vi "Save Results To Disk.vi"(0 "Save To Path":path, 1 "Sample Name":string, 2 "User Name":string, 3 "Test Date":string, 5 "Test Settings":T2={"Current Level"=0.0, "Compliance Level"=0.0, "Soak Time"=0.0, "NPLC Voltmeter"=1.0, "Count Voltmeter"=1, "NPLC Ammeter"=1.0, "Count Ammeter"=1, "Sample Resistivity"=enum."Low", "Sample Thickness"=0.0, "Magnetic Flux"=0.0, "Units"=enum."T", "Sample Dimensions x"=0.0, "Sample Dimensions y"=0.0, "Sample Dimensions D1"=0.0, "Sample Dimensions D2"=0.0, "Sample Width Ws"=0.0, "Slot Number of 3765 Card"=1} {"Slot Number of 3765 Card" min=1 max=6 step=1; "NPLC Ammeter" min=0.01 max=10.0; "NPLC Voltmeter" min=0.01 max=10.0 format="%^#_6g"; "Count Ammeter" min=1 max=1024; "Count Voltmeter" min=1 max=1024; "Soak Time" format="%^#_6g"; "Compliance Level" format="%^#_6g"; "Current Level" format="%^#_6e"}, 7 "Van Der Pauw Measurements":T5, 9 "Van Der Pauw Resistance Results":T3, 11 "error in (no error)":errorcluster, 12 "Hall Measurements":T5, 13 "Hall Effect Results":T4) -> (15 "error out":errorcluster)   [LabVIEW 2016]
uses:
  Hall Effect Library/Public/Controls/Resisitivity.ctl
  Hall Effect Library/Hall Effect Library.lvlib
panel:
  # "NPLC"
  # "A"
  # "V"
  # "s"
  # "Measure Count"
  # "cm"
  # "cm"
  # "cm"
  # "cm"
  # "cm"
  # "cm"
  # "Geometric Factor"
  # "Resistance Ratio"
  # "Resistivity"
  # "Ohm cm"
  # "Ohm cm"
  # "Ohm cm"
  # "Hall Coefficient"
  # "cm^2/V s"
  # "Ohm cm"
  # "cm^-3"
  # "Ohm cm"
  # "Ohm cm"
  # "Current"
  # "Pos"
  # "Volts"
  # "Neg"
  # "Direction"
  # "Magnet"
  # "Pos"
  # "Volts"
  # "Neg"
  # "Polarity"
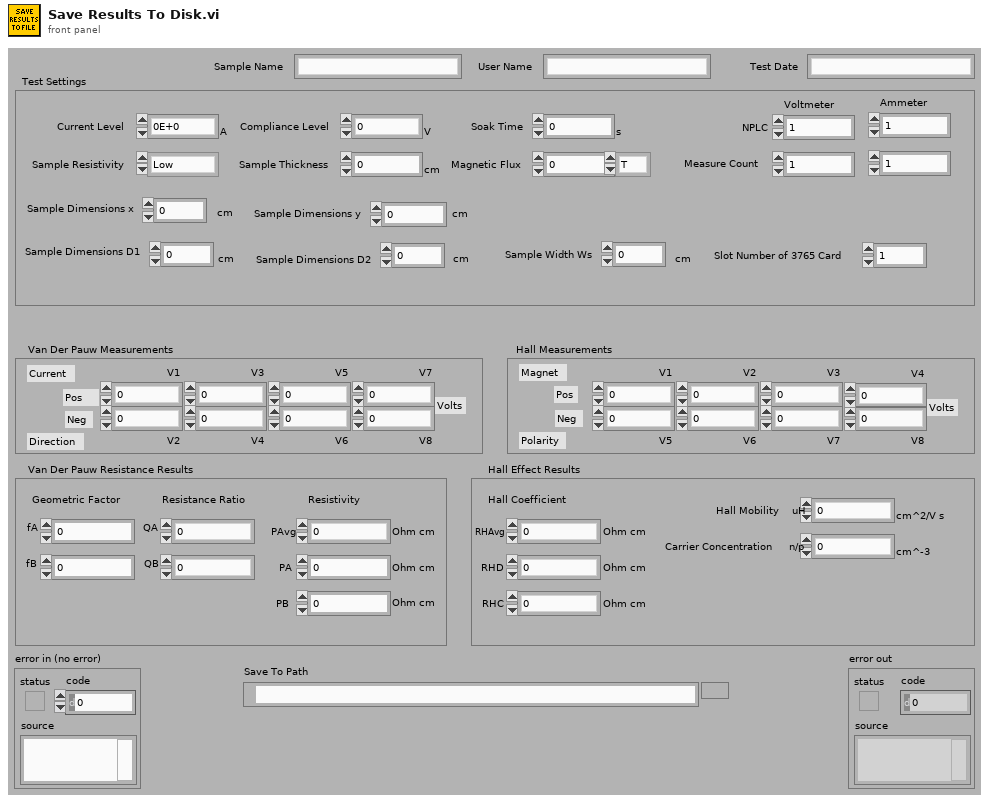
[diagram p1: front panel]
types:
  T1 = typedef "Hall Effect Library.lvlib/Resisitivity.ctl" = enum16{"Low", "High"}
  T2 = cluster{"Current Level":dbl, "Compliance Level":dbl, "Soak Time":dbl, "NPLC Voltmeter":dbl, "Count Voltmeter":i32, "NPLC Ammeter":dbl, "Count Ammeter":i32, "Sample Resistivity":T1, "Sample Thickness":dbl, "Magnetic Flux":dbl, "Units":enum16{"Gs", "T"}, "Sample Dimensions x":dbl, "Sample Dimensions y":dbl, "Sample Dimensions D1":dbl, "Sample Dimensions D2":dbl, "Sample Width Ws":dbl, "Slot Number of 3765 Card":u8}
  T3 = cluster{"fA":dbl, "fB":dbl, "QA":dbl, "QB":dbl, "PAvg":dbl, "PA":dbl, "PB":dbl}
  T4 = cluster{"RHD":dbl, "RHC":dbl, "RHAvg":dbl, "uH":dbl, "n/p":dbl}
  T5 = cluster{"V1":dbl, "V2":dbl, "V3":dbl, "V4":dbl, "V5":dbl, "V6":dbl, "V7":dbl, "V8":dbl}
  T6 = enum16{"open", "replace", "create", "open or create", "replace or create", "replace or create with confirmation"}
  T7 = cluster{"Van Der Pauw Currents[0]":dbl, "Van Der Pauw Currents[1]":dbl, "Van Der Pauw Currents[2]":dbl, "Van Der Pauw Currents[3]":dbl, "Van Der Pauw Currents[4]":dbl, "Van Der Pauw Currents[5]":dbl, "Van Der Pauw Currents[6]":dbl, "Van Der Pauw Currents[7]":dbl}
  T8 = cluster{"Hall Effect Currents[0]":dbl, "Hall Effect Currents[1]":dbl, "Hall Effect Currents[2]":dbl, "Hall Effect Currents[3]":dbl, "Hall Effect Currents[4]":dbl, "Hall Effect Currents[5]":dbl, "Hall Effect Currents[6]":dbl, "Hall Effect Currents[7]":dbl}
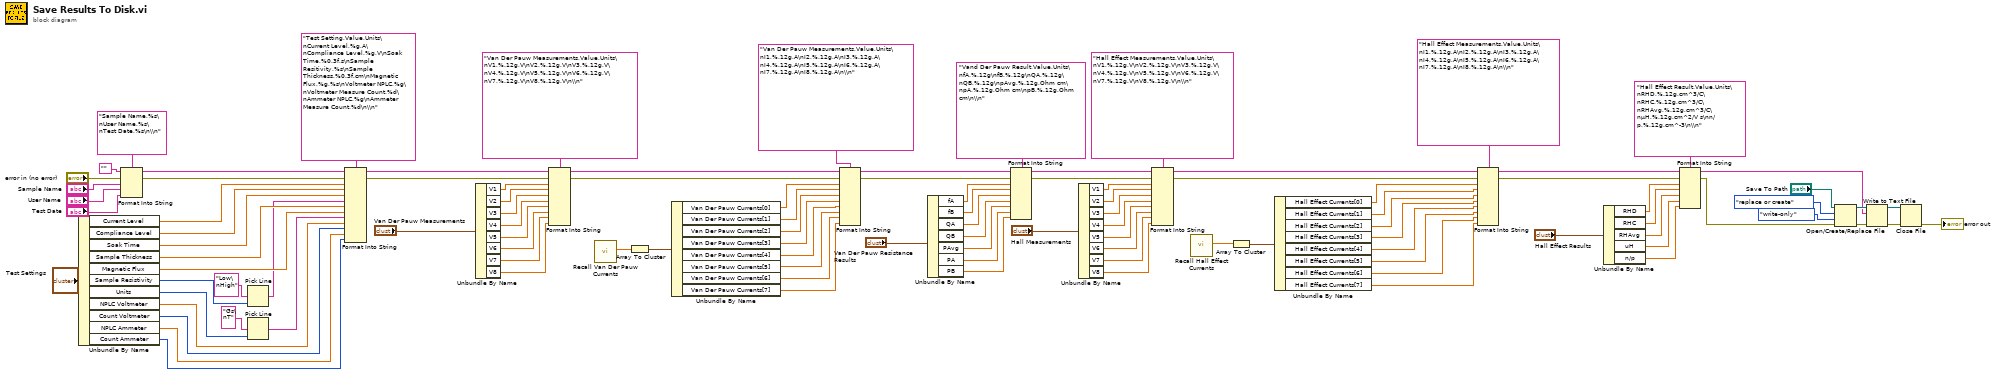
[diagram p0: block diagram]
diagram:
  n1 = Unbundle By Name("Test Settings") -> ("Current Level"=w98:dbl, "Compliance Level"=w97:dbl, "Soak Time"=w96:dbl, "Sample Thickness"=w95:dbl, "Magnetic Flux"=w94:dbl, "Sample Resistivity"=w90:T1, "Units"=w91:enum16{"Gs", "T"}, "NPLC Voltmeter"=w35:dbl, "Count Voltmeter"=w34:i32, "NPLC Ammeter"=w33:dbl, "Count Ammeter"=w32:i32)
  n2 = Format Into String(format string="Sample Name,%s\nUser Name,%s\nTest Date,%s\n\\n", initial string="", error in="error in (no error)", "Sample Name", "User Name", "Test Date") -> (resulting string=w86:string, error out=w87:errorcluster)
  n3 = Pick Line(multi-line string="Low\nHigh", line index=w90) -> (output string=w89:string)  [unwired: 1 out]
  n4 = Pick Line(multi-line string="Gs\nT", line index=w91) -> (output string=w88:string)  [unwired: 1 out]
  n5 = Format Into String(format string="Test Setting,Value,Units\nCurrent Level,%g,A\nCompliance Level,%g,V\nSoak Time,%0.3f,s\nSample Resitivity,%s\nSample Thickness,%0.3f,cm\nMagnetic Flux,%g,%s\nVoltmeter NPLC,%g\nVoltmeter Measure Count,%d\nAmmeter NPLC,%g\nAmmeter Measure Count,%d\n\\n", initial string=w86, error in=w87, w98, w97, w96, w89, w95, w94, w88, w35, w34, w33, w32) -> (resulting string=w83:string, error out=w82:errorcluster)
  n6 = Unbundle By Name("Van Der Pauw Measurements") -> ("V1"=w81:dbl, "V2"=w80:dbl, "V3"=w79:dbl, "V4"=w78:dbl, "V5"=w77:dbl, "V6"=w76:dbl, "V7"=w75:dbl, "V8"=w74:dbl)
  n7 = Format Into String(format string="Van Der Pauw Measurements,Value,Units\nV1,%.12g,V\nV2,%.12g,V\nV3,%.12g,V\nV4,%.12g,V\nV5,%.12g,V\nV6,%.12g,V\nV7,%.12g,V\nV8,%.12g,V\n\\n", initial string=w83, error in=w82, w81, w80, w79, w78, w77, w76, w75, w74) -> (resulting string=w28:string, error out=w27:errorcluster)
  n8 = call "Recall Van Der Pauw Currents.vi"() -> ("Van Der Pauw Currents"=w30:dbl[])  [unwired: 11 in]
  n9 = Array To Cluster(array=w30) -> (cluster=w29:T7)
  n10 = Unbundle By Name(w29) -> ("Van Der Pauw Currents[0]"=w26:dbl, "Van Der Pauw Currents[1]"=w25:dbl, "Van Der Pauw Currents[2]"=w24:dbl, "Van Der Pauw Currents[3]"=w23:dbl, "Van Der Pauw Currents[4]"=w22:dbl, "Van Der Pauw Currents[5]"=w21:dbl, "Van Der Pauw Currents[6]"=w20:dbl, "Van Der Pauw Currents[7]"=w19:dbl)
  n11 = Format Into String(format string="Van Der Pauw Measurements,Value,Units\nI1,%.12g,A\nI2,%.12g,A\nI3,%.12g,A\nI4,%.12g,A\nI5,%.12g,A\nI6,%.12g,A\nI7,%.12g,A\nI8,%.12g,A\n\\n", initial string=w28, error in=w27, w26, w25, w24, w23, w22, w21, w20, w19) -> (resulting string=w17:string, error out=w16:errorcluster)
  n12 = Unbundle By Name("Van Der Pauw Resistance Results") -> ("fA"=w62:dbl, "fB"=w61:dbl, "QA"=w60:dbl, "QB"=w59:dbl, "PAvg"=w58:dbl, "PA"=w57:dbl, "PB"=w56:dbl)
  n13 = Format Into String(format string="Vand Der Pauw Result,Value,Units\nfA,%.12g\nfB,%.12g\nQA,%.12g\nQB,%.12g\npAvg,%.12g,Ohm cm\npA,%.12g,Ohm cm\npB,%.12g,Ohm cm\n\\n", initial string=w17, error in=w16, w62, w61, w60, w59, w58, w57, w56) -> (resulting string=w55:string, error out=w54:errorcluster)
  n14 = Unbundle By Name("Hall Measurements") -> ("V1"=w66:dbl, "V2"=w67:dbl, "V3"=w68:dbl, "V4"=w69:dbl, "V5"=w70:dbl, "V6"=w71:dbl, "V7"=w72:dbl, "V8"=w73:dbl)
  n15 = Format Into String(format string="Hall Effect Measurements,Value,Units\nV1,%.12g,V\nV2,%.12g,V\nV3,%.12g,V\nV4,%.12g,V\nV5,%.12g,V\nV6,%.12g,V\nV7,%.12g,V\nV8,%.12g,V\n\\n", initial string=w55, error in=w54, w66, w67, w68, w69, w70, w71, w72, w73) -> (resulting string=w13:string, error out=w12:errorcluster)
  n16 = call "Recall Hall Effect Currents.vi"() -> ("Hall Effect Currents"=w15:dbl[])  [unwired: 11 in]
  n17 = Array To Cluster(array=w15) -> (cluster=w14:T8)
  n18 = Unbundle By Name(w14) -> ("Hall Effect Currents[0]"=w11:dbl, "Hall Effect Currents[1]"=w10:dbl, "Hall Effect Currents[2]"=w9:dbl, "Hall Effect Currents[3]"=w8:dbl, "Hall Effect Currents[4]"=w7:dbl, "Hall Effect Currents[5]"=w6:dbl, "Hall Effect Currents[6]"=w5:dbl, "Hall Effect Currents[7]"=w4:dbl)
  n19 = Format Into String(format string="Hall Effect Measurements,Value,Units\nI1,%.12g,A\nI2,%.12g,A\nI3,%.12g,A\nI4,%.12g,A\nI5,%.12g,A\nI6,%.12g,A\nI7,%.12g,A\nI8,%.12g,A\n\\n", initial string=w13, error in=w12, w11, w10, w9, w8, w7, w6, w5, w4) -> (resulting string=w3:string, error out=w2:errorcluster)
  n20 = Unbundle By Name("Hall Effect Results") -> ("RHD"=w51:dbl, "RHC"=w50:dbl, "RHAvg"=w49:dbl, "uH"=w48:dbl, "n/p"=w47:dbl)
  n21 = Format Into String(format string="Hall Effect Result,Value,Units\nRHD,%.12g,cm^3/C\nRHC,%.12g,cm^3/C\nRHAvg,%.12g,cm^3/C\nµH,%.12g,cm^2/V s\nn/p,%.12g,cm^-3\n\\n", initial string=w3, error in=w2, w51, w50, w49, w48, w47) -> (resulting string=w38:string, error out=w39:errorcluster)
  n22 = Open/Create/Replace File(file path (use dialog)="Save To Path", error in=w39, operation (0:open)=T6."replace or create", access (0:read/write)=enum16{"read/write", "read-only", "write-only"}."write-only") -> (refnum out=w43:refnum<file>, error out=w42:errorcluster)  [unwired: 3 out]
  n23 = Write to Text File(file (use dialog)=w43, text=w38, error in=w42) -> (refnum out=w40:refnum<file>, error out=w41:errorcluster)  [unwired: 2 out]
  n24 = Close File(refnum=w40, error in=w41) -> (error out=→"error out":errorcluster)  [unwired: 1 out]
